vi "Benchmark - LabVIEW vs SharedLib.vi"() -> ()   [LabVIEW 2023]
uses:
  <vilib>/Analysis/1siggen.llb/Ramp Pattern by Samples.vi
  4685aa10-b952-4efc-93a5-7bd3492d3515.vi
  4685aa10-b952-4efc-93a5-7bd3492d3515.vi/5f8c2839-cca9-114a-b070-6418e2096687.vi
  4685aa10-b952-4efc-93a5-7bd3492d3515.vi/903ae9db-7fdb-7945-9162-e2f51a82b5df.vi
  4685aa10-b952-4efc-93a5-7bd3492d3515.vi/c538dc2b-b02a-fe43-8866-95cbc1854757.vi
  4685aa10-b952-4efc-93a5-7bd3492d3515.vi/bc4324fb-7fbb-b448-adb0-52943a190b69.vi
  4685aa10-b952-4efc-93a5-7bd3492d3515.vi/bb695ee8-a326-0b45-aed1-b7b7f3896d70.vi
  <vilib>/picture/picture.llb/Draw True-Color Pixmap.vi
  <vilib>/Analysis/NI_AALBase.lvlib
panel:
  in  "gamma (1,9)":dbl=1.9 format="%#_13g"
  out "Threads":i32
  out "Pix.":i32
  out "Ratio":dbl=inf format="%.1f"
  in  "Scale (8)":i32=512
  out "result\nPASS":bool
  out "ns/pixel (dll)":dbl format="%.2f"
  out "DLL, ms":u32
  out "2D Picture":picture
  out "ns/pixel (ref)":dbl format="%.2f"
  out "Rows (Height)":i32
  out "Cols (Width)":i32
  out "LabVIEW, ms":u32
  # "The DLL was built using Microsoft Visual Studio 2022 compiler\n\nTo open execute this VI you may need to download and install\nMicrosoft Visual C++ Redistributable\nhttps://learn.microsoft.com/en-us/cpp/windows/latest-supported-vc-redist?view=msvc-170"
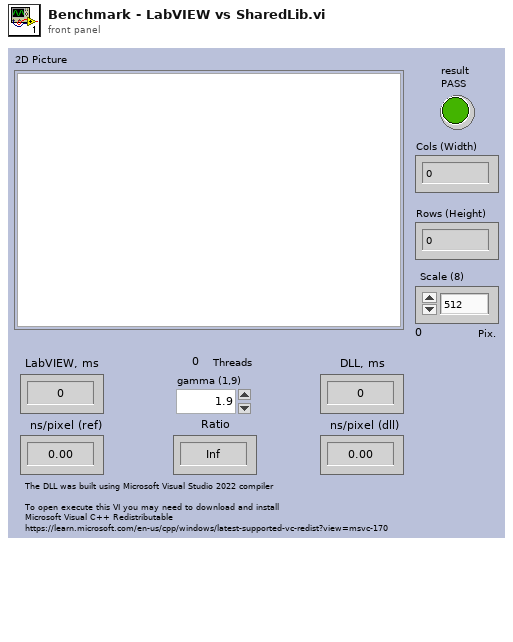
[diagram p1: front panel]
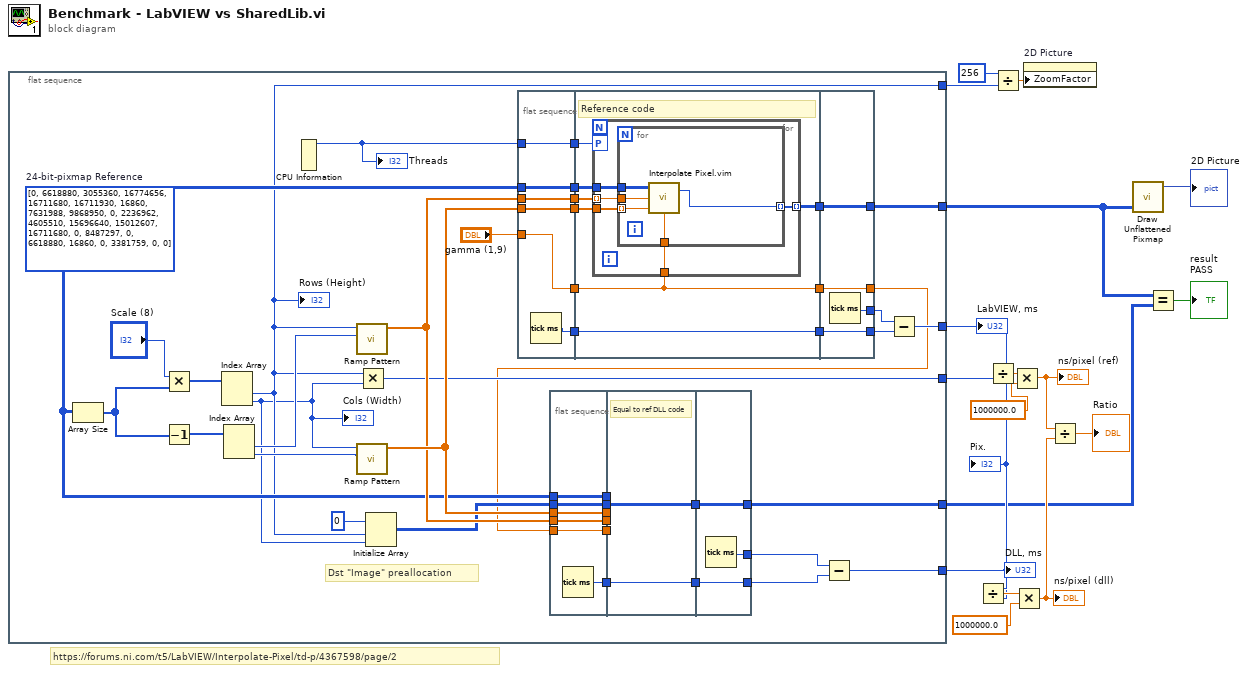
[diagram p0: block diagram]
diagram:
  # "https://forums.ni.com/t5/LabVIEW/Interpolate-Pixel/td-p/4367598/page/2"
  n1 = flat-sequence {
    tunnel: [w53] -> w2
    tunnel: [w42] -> w1
    tunnel: [w24] -> w14
    tunnel: [w25] -> w6
    tunnel: [w32] -> w12
    tunnel: [w29] -> w4
    frame #0 {
      w39 = u32[][] [[0, 6618880, 3055360, 16774656, 16711680, 16711930], [16860, 7631988, 9868950, 0, 2236962, 4605510], [15696640, 15012607, 16711680, 0, 8487297, 0], [6618880, 16860, 0, 3381759, 0, 0]]  # 24-bit-pixmap Reference
      # "Dst \"Image\" preallocation"
      n2 = Array Size(array=w39) -> (size(s)=w58:i32[])
      n3 = Multiply(x="Scale (8)", y=w58) -> (x*y=w56:i32[])
      n4 = Decrement(x=w58) -> (x-1=w57:i32[])
      n5 = Index Array(array=w56) -> (element #1=w29:i32, element #2=w28:i32)  [unwired: 2 in]
      "Cols (Width)" <- w28
      "Rows (Height)" <- w29
      n6 = Index Array(array=w57) -> (element #1=w54:i32, element #2=w55:i32)  [unwired: 2 in]
      n7 = CPU Information() -> (4:w23:i32)  [unwired: 3 out]
      "Threads" <- w23
      n8 = call-poly <vilib>:"Ramp Pattern.vi"("end"=w54, "samples"=w29) -> ("Ramp Pattern"=w40:dbl[])  [unwired: 8 in, 1 out]
      n9 = call-poly <vilib>:"Ramp Pattern.vi"("end"=w55, "samples"=w28) -> ("Ramp Pattern"=w43:dbl[])  [unwired: 8 in, 1 out]
      n10 = Multiply(x=w29, y=w28) -> (x*y=w25:i32)
      n11 = Initialize Array(u32 0 ("return type"), w29, w28) -> (w26:u32[][])
      n12 = flat-sequence {
        tunnel: w43 -> [w74]
        tunnel: w40 -> [w75]
        tunnel: w39 -> [w76]
        tunnel: [w76] -> w52
        tunnel: [w75] -> w51
        tunnel: [w74] -> w50
        tunnel: [w73] -> w36
        tunnel: [w72] -> w31
        tunnel: w23 -> [w72]
        tunnel: [w71] -> w22
        tunnel: "gamma (1,9)" -> [w71]
        tunnel: w52 -> [w83]
        tunnel: w51 -> [w82]
        tunnel: w50 -> [w81]
        tunnel: [w80] -> w49
        tunnel: [w79] -> w37
        tunnel: w36 -> [w79]
        tunnel: w31 -> [w78]
        tunnel: w22 -> [w77]
        tunnel: [w77] -> w18
        tunnel: [w97] -> w53
        tunnel: w49 -> [w97]
        tunnel: [w96] -> w48
        tunnel: [w95] -> w38
        tunnel: w37 -> [w95]
        tunnel: [w94] -> w19
        tunnel: w18 -> [w94]
        frame #0 {
          n13 = Tick Count (ms)() -> (millisecond timer value=w73:u32)
        }
        frame #1 {
          # "Reference code"
          n14 = for {
            tunnel: w83 -> [w88]
            tunnel: w82 -> [w87] mode=indexing
            tunnel: w81 -> [w86]
            tunnel: [w85] -> w80 mode=indexing
            workers-P: w78 -> [_]
            tunnel: w77 -> [w84]
            n15 = for {
              tunnel: w88 -> [w93]
              tunnel: w87 -> [w92]
              tunnel: w86 -> [w91] mode=indexing
              tunnel: [w90] -> w85 mode=indexing
              tunnel: w84 -> [w89]
              n16 = call "Interpolate Pixel.vim"("gamma"=w89, "Fractional Column"=w91, "Fractional Row"=w92, "24-bit PixMap"=w93) -> ("Pixel Value"=w90:u32)  [unwired: 1 in]
            }
          }
        }
        frame #2 {
          n17 = Tick Count (ms)() -> (millisecond timer value=w96:u32)
        }
      }
      n18 = flat-sequence {
        tunnel: w43 -> [w63]
        tunnel: w40 -> [w64]
        tunnel: w39 -> [w65]
        tunnel: [w65] -> w47
        tunnel: [w64] -> w46
        tunnel: [w63] -> w45
        tunnel: [w62] -> w35
        tunnel: [w61] -> w27
        tunnel: w26 -> [w61]
        tunnel: [w60] -> w20
        tunnel: w19 -> [w60]
        tunnel: w47 -> [_]
        tunnel: w46 -> [_]
        tunnel: w45 -> [_]
        tunnel: [w66] -> w44
        tunnel: w35 -> [w67]
        tunnel: [w67] -> w34
        tunnel: w27 -> [w66]
        tunnel: w20 -> [_]
        tunnel: [w70] -> w42
        tunnel: w44 -> [w70]
        tunnel: [w69] -> w41
        tunnel: w34 -> [w68]
        tunnel: [w68] -> w33
        frame #0 {
          n19 = Tick Count (ms)() -> (millisecond timer value=w62:u32)
        }
        frame #1 {
          # "Equal to ref DLL code"
        }
        frame #2 {
          n20 = Tick Count (ms)() -> (millisecond timer value=w69:u32)
        }
      }
      n21 = Subtract(x=w41, y=w33) -> (x-y=w32:u32)
      n22 = Subtract(x=w48, y=w38) -> (x-y=w24:u32)
    }
  }
  n23 = Divide(x=w12, y=w6) -> (x/y=w13:dbl)
  n24 = Divide(x=w14, y=w6) -> (x/y=w16:dbl)
  n25 = Divide(x=256, y=w4) -> (x/y=w3:dbl)
  n26 = Multiply(x=w16, y=1000000.0) -> (x*y=w10:dbl)
  "ns/pixel (ref)" <- w10
  n27 = Multiply(x=w13, y=1000000.0) -> (x*y=w9:dbl)
  "ns/pixel (dll)" <- w9
  n28 = property on="2D Picture" class="Pict"("ZoomFactor"=w3) -> ()  [unwired: 2 in, 2 out]
  n29 = Divide(x=w10, y=w9) -> (x/y=→"Ratio":dbl)
  n30 = call-poly <vilib>:"Draw Unflattened Pixmap.vi"("data (RGB format)"=w2) -> ("new picture"=→"2D Picture":picture)  [unwired: 8 in]
  n31 = Equal?(x=w2, y=w1) -> (x = y?=→"result\nPASS":bool)
  "LabVIEW, ms" <- w14
  "DLL, ms" <- w12
  "Pix." <- w6
